vi "SW_Generate_Segmented_Plot_v2.vi"(0 "Draw Area Size":cluster{"Width":dbl, "Height":dbl}={"Width"=480.0, "Height"=480.0}, 1 "Input cluster of parameters":T1={"Amount of border segments"=8, "Border segments starting angle"=0, "Amount of midfield segments"=4, "Midfield segments starting angle"=0, "Midfield segments outer radius, mm"=60, "Amount of central segments"=1, "Center segment outer radius, mm"=30}, 2 "Diameter of the cage, mm":u16(knob)=180 scale=20.0..250.0, 3 "R-gap between segments, mm":u8=10, 4 "Colors array for outer segments":u32[](array[numeric])=[14102567, 16625249, 14742520, 7646673, 16018755, 16703632, 11262441, 4552116], 5 "Error In":errorcluster, 6 "Regions to mark":u16[](array[numeric]), 7 "Colors array for midfield segments":u32[](array[numeric])=[8073876, 10935200, 34871, 12756431], 9 "Color for central segment":u32=16777113) -> (12 "No zones Display output":picture, 14 "Zones Display output":picture, 15 "Actual parameters output":T4, 16 "Array of the segment to color correspondences":u32[][](array[numeric]), 17 "Array of the pixel to color correspondences":u32[][](array[numeric]), 18 "Pixels per mm":dbl=2.533333333333333, 19 "Error Out":errorcluster)   [LabVIEW 2016]
panel:
  out "Fonts scale factor":dbl
  out "Coordinates of the center of the image":T2
  out "Center segments outer radius, pix":dbl
  out "Midfield segments outer radius, pix":dbl
  out "Bounding rectangle of the midfield segments":T3
  out "Bounding rectangle for outer segments":T3
  in  "Fill color for no segments image":u32(colorbox)=6316128
  out "Radius of displayed outer segments, pix":dbl=228.0
  in  "Background color":u32(colorbox)=13816530
  in  "Zones Display input":picture
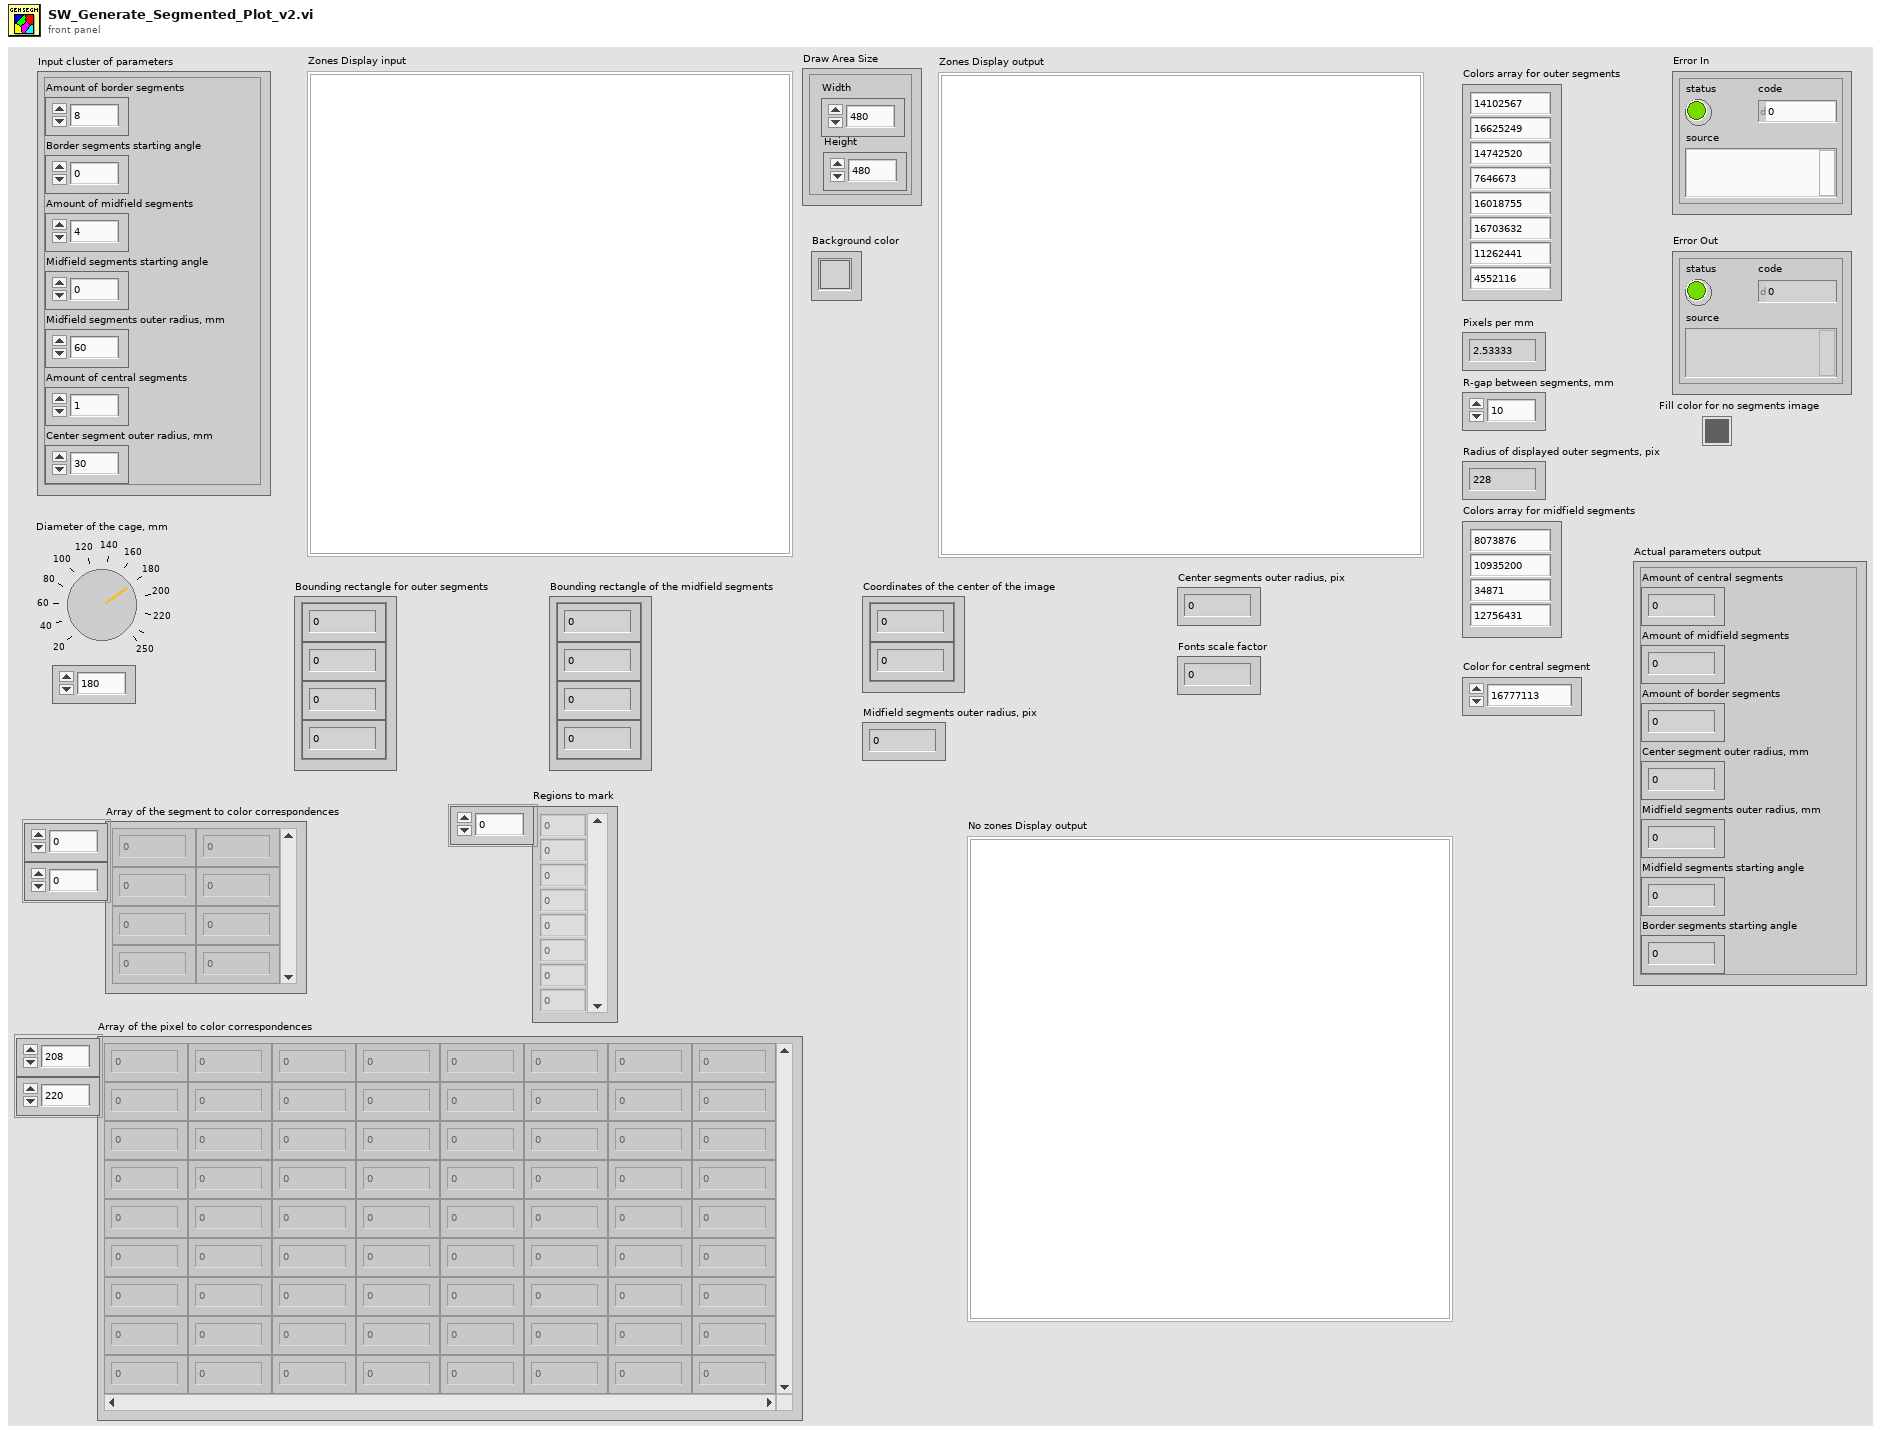
[diagram p1: front panel]
types:
  T1 = cluster{"Amount of border segments":u8, "Border segments starting angle":i16, "Amount of midfield segments":u8, "Midfield segments starting angle":i16, "Midfield segments outer radius, mm":u16, "Amount of central segments":u8, "Center segment outer radius, mm":u16}
  T2 = cluster{"Numeric Control":dbl, "Numeric Control":dbl}
  T3 = cluster{"Numeric Control":dbl, "Numeric Control":dbl, "Numeric Control":dbl, "Numeric Control":dbl}
  T4 = cluster{"Amount of central segments":u8, "Amount of midfield segments":u8, "Amount of border segments":u8, "Center segment outer radius, mm":u16, "Midfield segments outer radius, mm":u16, "Midfield segments starting angle":i16, "Border segments starting angle":i16}
  T5 = enum16{"User-specified Font", "Application Font", "System Font", "Dialog Font"}
  T6 = cluster{"horizontal":enum16{"left", "center", "right"}, "vertical":enum16{"top", "center", "bottom"}}
  T7 = cluster{"Width":u16, "Style":enum32{"Solid", "Dash", "Dot", "DashDot", "DashDotDot"}}
  T8 = cluster{"Amount of central segments":u8, "Amount of midfield segments":u8, "Amount of border segments":u8, u16, u16, i16, i16}
  T9 = typedef "imagedata.ctl" = cluster{"image type":i32, "image depth":i32, "image":u8[], "mask":u8[], "colors":u32[], "Rectangle":cluster{"left":i16, "top":i16, "right":i16, "bottom":i16}}
  T10 = cluster{"left":i16, "top":i16, "right":i16, "bottom":i16}
  T11 = cluster{"image[0]":u8, "image[1]":u8, "image[2]":u8}
  T12 = cluster{"Font Name:":string, "Size":i16, "Strikeout?":bool, "Italic?":bool, "Underline?":bool, "Outline?":bool, "Shadow?":bool, "Bold?":bool}
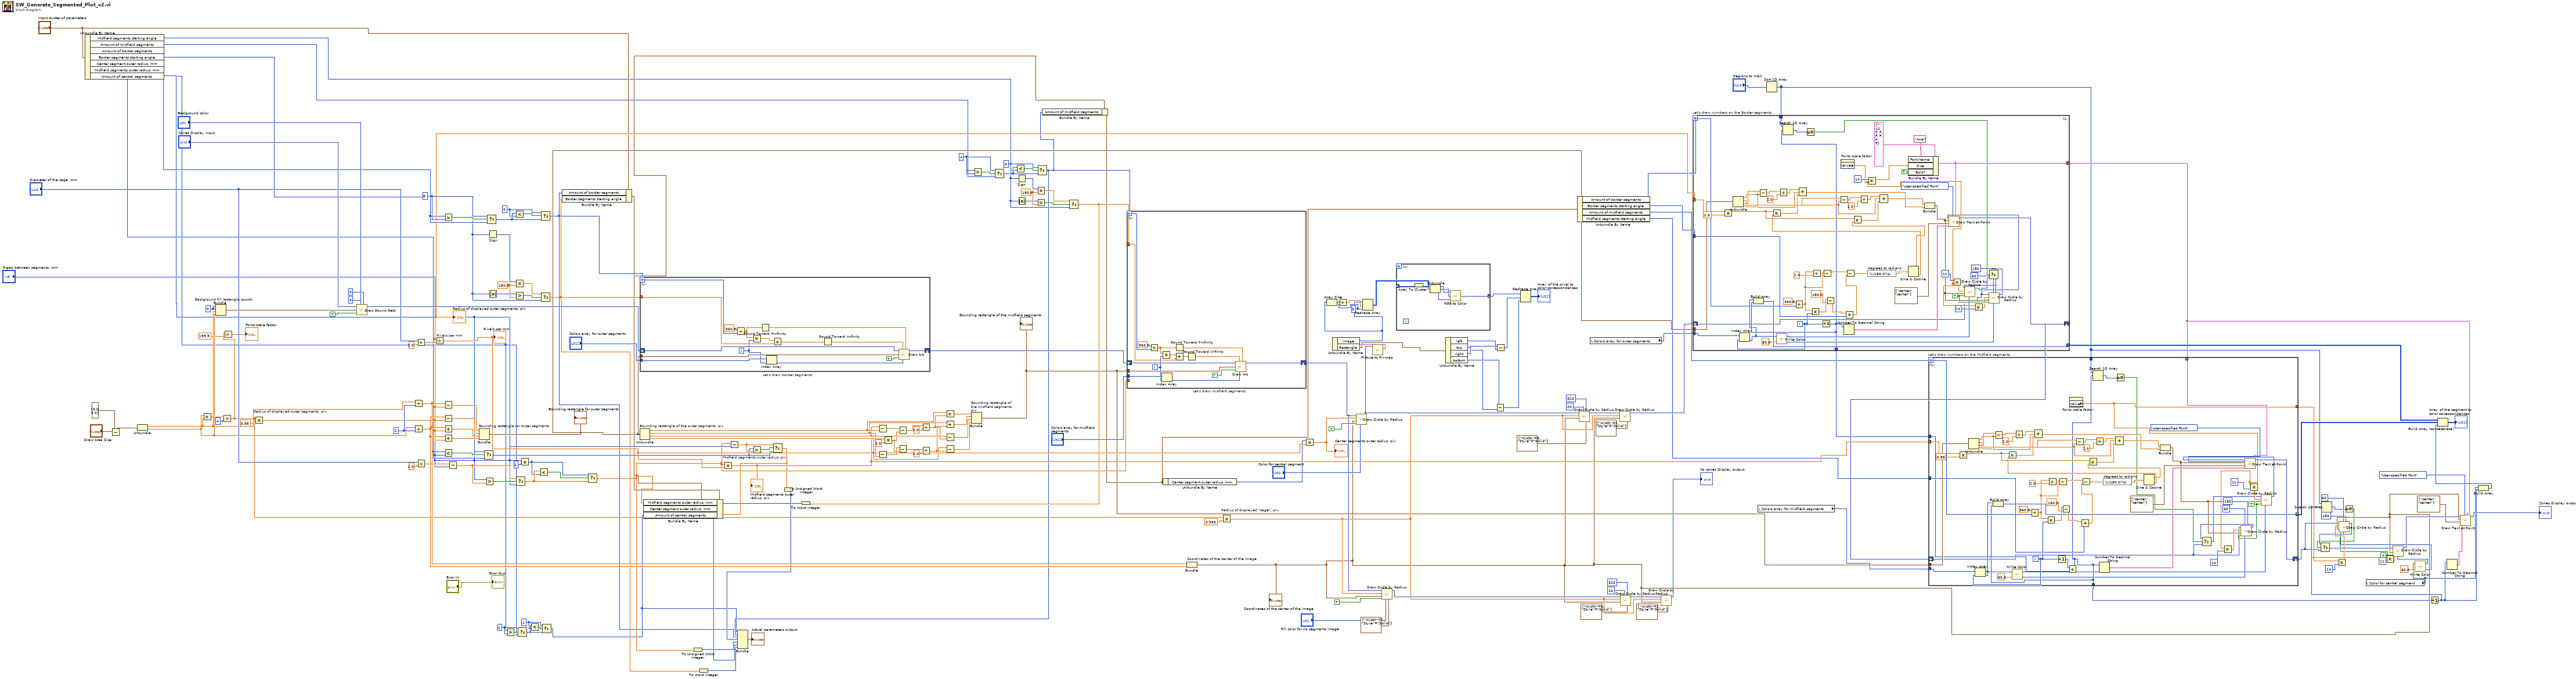
[diagram p0: block diagram]
diagram:
  w59 = 3 ("dimension size")
  w5 = TRUE ("fill?(F)")
  w146 = 180.0 ("y")
  w152 = u8 1 ("y")
  w149 = u8 1 ("y")
  w153 = u8 4 ("y")
  w156 = u8 0 ("y")
  w176 = u8 0 ("y")
  w178 = u8 8 ("y")
  w181 = 180.0 ("y")
  w190 = u32 2 ("y")
  w192 = 0
  n1 = Unbundle By Name("Input cluster of parameters") -> ("Midfield segments starting angle"=w29:i16, "Amount of midfield segments"=w28:u8, "Amount of border segments"=w27:u8, "Border segments starting angle"=w26:i16, "Center segment outer radius, mm"=w25:u16, "Midfield segments outer radius, mm"=w24:u16, "Amount of central segments"=w23:u8)
  n2 = Subtract(x="Draw Area Size", y=cluster{"Width":dbl, "Height":dbl} {"Width"=6.0, "Height"=6.0}) -> (x-y=w87:cluster{"Width":dbl, "Height":dbl})
  n3 = Unbundle(w87) -> ("Width"=w188:dbl, "Height"=w189:dbl)
  n4 = Add(x=w189, y=w188) -> (x+y=w187:dbl)
  n5 = Bundle "Background fill rectangle coords"(w192, w192, "Width"=w188, "Height"=w189) -> (w174:cluster{i32, i32, "Width":dbl, "Height":dbl})  [unwired: 1 in]
  n6 = Divide(x=w187, y=u32 4) -> (x/y=w22:dbl)
  n7 = Divide(x=w22, y=199.5) -> (x/y=→"Fonts scale factor":dbl)
  n8 = Multiply "Radius of displayed outer segments, pix"(x=w22, y=0.95) -> (x*y=w71:dbl)
  "Radius of displayed outer segments, pix" <- w71
  n9 = call <vilib>:"Draw Round Rect.vi"("picture"="Zones Display input", "oval width"=i16 0, "rect"=w174, "fill?(F)"=TRUE, "color(black)"="Background color", "oval height"=i16 0) -> ("new picture"=w173:picture)  [unwired: 3 in]
  n10 = Divide(x=w188, y=w190) -> (x/y=w172:dbl)
  n11 = Divide(x=w189, y=w190) -> (x/y=w171:dbl)
  n12 = Divide(x="Diameter of the cage, mm", y=2.0) -> (x/y=w160:dbl)
  n13 = Divide(x="Diameter of the cage, mm", y=2.0) -> (x/y=w138:dbl)
  n14 = Divide "Pixels per mm"(x=w71, y=w160) -> (x/y=w100:dbl)
  "Pixels per mm" <- w100
  n15 = Greater?(x=w27, y=w178) -> (0:w179:bool)
  n16 = Subtract(x=w172, y=w71) -> (x-y=w170:dbl)
  n17 = Subtract(x=w171, y=w71) -> (x-y=w169:dbl)
  n18 = Add(x=w172, y=w71) -> (x+y=w168:dbl)
  n19 = Add(x=w171, y=w71) -> (x+y=w167:dbl)
  n20 = Less?(x=w25, y="R-gap between segments, mm") -> (x < y?=w136:bool)
  n21 = Subtract(x=w138, y="R-gap between segments, mm") -> (x-y=w141:dbl)
  n22 = Bundle "Bounding rectangle for outer segments"(w170, w169, w168, w167) -> (w72:cluster{dbl, dbl, dbl, dbl})  [unwired: 1 in]
  "Bounding rectangle for outer segments" <- w72
  n23 = Select(t="R-gap between segments, mm", s=w136, f=w25) -> (s? t:f=w133:u16)
  n24 = Greater?(x=w24, y=w141) -> (0:w142:bool)
  n25 = Select(t=w178, s=w179, f=w27) -> (s? t:f=w175:u8)
  n26 = Sign(1:w26) -> (0:w182:i16)
  n27 = Absolute Value(x=w26) -> (abs(x)=w184:i16)
  n28 = Greater?(x=w23, y=w152) -> (0:w151:bool)
  n29 = Less?(x=w175, y=w176) -> (x < y?=w177:bool)
  n30 = Multiply(x=w182, y=w181) -> (x*y=w180:dbl)
  n31 = Greater?(x=w184, y=w181) -> (0:w183:bool)
  n32 = Select(t=w141, s=w142, f=w24) -> (s? t:f=w139:dbl)
  n33 = Select(t=w152, s=w151, f=w23) -> (s? t:f=w148:u8)
  n34 = Multiply(x="R-gap between segments, mm", y=u8 2) -> (x*y=w132:u8)
  n35 = Less?(x=w148, y=w149) -> (x < y?=w150:bool)
  n36 = Less?(x=w139, y=w132) -> (x < y?=w140:bool)
  n37 = Select(t=w176, s=w177, f=w175) -> (s? t:f=w44:u8)
  n38 = Select(t=w180, s=w183, f=w26) -> (s? t:f=w43:dbl)
  n39 = Select(t=w149, s=w150, f=w148) -> (s? t:f=w37:u8)
  n40 = Bundle By Name(cluster="Input cluster of parameters", "Amount of border segments"=w44, "Border segments starting angle"=w43) -> (w41:T1)
  n41 = Select(t=w132, s=w140, f=w139) -> (s? t:f=w39:dbl)
  n42 = for "Let's draw border segments" {
    N: w44 -> [w203]
    tunnel: w43 -> [w208]
    shift-right: [w201] -> w158
    shift-left: w173 -> [w210]
    tunnel: w72 -> [w204]
    tunnel: "Colors array for outer segments" -> [w207]
    i -> [w198]
    n43 = Divide(x=360.0, y=w203) -> (x/y=w202:dbl)
    n44 = Multiply(x=w202, y=w198) -> (x*y=w209:dbl)
    n45 = Round Toward +Infinity(x=w202) -> (ceil(x): smallest int >= x=w200:dbl)
    n46 = Index Array(array=w207, index=w198) -> (element=w197:u32)
    n47 = Add(x=w209, y=w208) -> (x+y=w205:dbl)
    n48 = Round Toward -Infinity(1:w205) -> (0:w199:dbl)
    n49 = call <vilib>:"Draw Arc.vi"("picture"=w210, "start angle[degrees]"=w199, "rect"=w204, "fill?(F)"=TRUE, "color(black)"=w197, "arc size[degrees]"=w200) -> ("new picture"=w201:picture)  [unwired: 3 in]
  }
  n50 = Unbundle "Bounding rectangle of the outer segments, pix"(w72) -> (w126:dbl, w118:dbl, w124:dbl, w117:dbl)
  n51 = To Unsigned Word Integer(number=w39) -> (unsigned 16bit integer=w105:u16)
  n52 = To Word Integer(number=w43) -> (16bit integer=w101:i16)
  n53 = Multiply "Midfield segments outer radius, pix"(x=w39, y=w100) -> (x*y=w69:dbl)
  "Midfield segments outer radius, pix" <- w69
  n54 = Subtract(x=w39, y="R-gap between segments, mm") -> (x-y=w134:dbl)
  n55 = Greater?(x=w133, y=w134) -> (0:w135:bool)
  n56 = Select(t=w134, s=w135, f=w133) -> (s? t:f=w38:dbl)
  n57 = Bundle By Name(cluster=w41, "Midfield segments outer radius, mm"=w39, "Center segment outer radius, mm"=w38, "Amount of central segments"=w37) -> (w40:T1)
  n58 = To Unsigned Word Integer(number=w38) -> (unsigned 16bit integer=w103:u16)
  n59 = Subtract(x=w124, y=w126) -> (x-y=w130:dbl)
  n60 = Subtract(x=w117, y=w118) -> (x-y=w123:dbl)
  n61 = Multiply(x=w69, y=2.0) -> (x*y=w122:dbl)
  n62 = Subtract(x=w130, y=w122) -> (x-y=w128:dbl)
  n63 = Subtract(x=w123, y=w122) -> (x-y=w120:dbl)
  n64 = Divide(x=w128, y=2.0) -> (x/y=w125:dbl)
  n65 = Divide(x=w120, y=2.0) -> (x/y=w119:dbl)
  n66 = Add(x=w126, y=w125) -> (x+y=w116:dbl)
  n67 = Add(x=w118, y=w119) -> (x+y=w114:dbl)
  n68 = Subtract(x=w124, y=w125) -> (x-y=w115:dbl)
  n69 = Subtract(x=w117, y=w119) -> (x-y=w113:dbl)
  n70 = Bundle "Bounding rectangle of the midfield segments, pix"(w116, w114, w115, w113) -> (w70:cluster{dbl, dbl, dbl, dbl})  [unwired: 1 in]
  "Bounding rectangle of the midfield segments" <- w70
  n71 = Greater?(x=w28, y=w153) -> (0:w154:bool)
  n72 = Select(t=w153, s=w154, f=w28) -> (s? t:f=w157:u8)
  n73 = Less?(x=w157, y=w156) -> (x < y?=w155:bool)
  n74 = Sign(1:w29) -> (0:w145:i16)
  n75 = Absolute Value(x=w29) -> (abs(x)=w143:i16)
  n76 = Multiply(x=w145, y=w146) -> (x*y=w147:dbl)
  n77 = Greater?(x=w143, y=w146) -> (0:w144:bool)
  n78 = Select(t=w156, s=w155, f=w157) -> (s? t:f=w42:u8)
  n79 = Bundle By Name(cluster=w40, "Amount of midfield segments"=w42) -> (w35:T1)
  n80 = Select(t=w147, s=w144, f=w29) -> (s? t:f=w104:dbl)
  n81 = To Word Integer(number=w104) -> (16bit integer=w102:i16)
  n82 = Bundle("Amount of central segments"=w37, "Amount of midfield segments"=w42, "Amount of border segments"=w44, w103, w105, w102, w101) -> (→"Actual parameters output":T8)  [unwired: 1 in]
  n83 = for "Let's draw midfield segments" {
    N: w42 -> [w217]
    shift-right: [w212] -> w93
    shift-left: w158 -> [w213]
    tunnel: w104 -> [w215]
    tunnel: w39 -> [_]
    tunnel: w70 -> [w214]
    tunnel: "Colors array for midfield segments" -> [w219]
    i -> [w216]
    n84 = Divide(x=360.0, y=w217) -> (x/y=w221:dbl)
    n85 = Multiply(x=w221, y=w216) -> (x*y=w222:dbl)
    n86 = Index Array(array=w219, index=w216) -> (element=w218:u32)
    n87 = Round Toward +Infinity(x=w221) -> (ceil(x): smallest int >= x=w224:dbl)
    n88 = Add(x=w222, y=w215) -> (x+y=w223:dbl)
    n89 = Round Toward -Infinity(1:w223) -> (0:w225:dbl)
    n90 = call <vilib>:"Draw Arc.vi"("picture"=w213, "start angle[degrees]"=w225, "rect"=w214, "fill?(F)"=TRUE, "color(black)"=w218, "arc size[degrees]"=w224) -> ("new picture"=w212:picture)  [unwired: 3 in]
  }
  n91 = Unbundle By Name(w35) -> ("Center segment outer radius, mm"=w36:u16)
  n92 = Bundle "Coordinates of the center of the image"(w172, w171) -> (w9:cluster{dbl, dbl})  [unwired: 1 in]
  "Coordinates of the center of the image" <- w9
  n93 = Multiply "Radius of displayed \"cage\", pix"(x=w22, y=0.955) -> (x*y=w89:dbl)
  n94 = Multiply(x=w36, y=w100) -> (x*y=w109:dbl)
  "Center segments outer radius, pix" <- w109
  n95 = call <vilib>:"Draw Circle by Radius.vi"("color(black)"="Color for central segment", "fill?(F)"=TRUE, "pixel center"=w9, "radius"=w109, "picture"=w93) -> ("new picture"=w63:picture)  [unwired: 6 in]
  n96 = call <vilib>:"Picture to Pixmap.vi"("picture"=w63) -> ("image data"=w62:T9)  [unwired: 9 in, 1 out]
  n97 = Unbundle By Name(w62) -> ("image"=w61:u8[], "Rectangle"=w56:T10)
  n98 = Array Size(array=w61) -> (size(s)=w60:i32)
  n99 = Divide(x=w60, y=w59) -> (x/y=w58:dbl)
  n100 = Reshape Array(w61, w58, w59) -> (w57:u8[][])
  n101 = call <vilib>:"Draw Circle by Radius.vi"("pen"=T7 {"Width"=2, "Style"=enum."Solid"}, "color(black)"="Fill color for no segments image", "fill?(F)"=TRUE, "pixel center"=w9, "radius"=w89, "picture"=w93) -> ("new picture"=w90:picture)  [unwired: 5 in]
  n102 = for {
    tunnel: w57 -> [w232] mode=indexing
    tunnel: [w227] -> w55 mode=indexing
    n103 = Array To Cluster(array=w232) -> (cluster=w231:T11)
    n104 = Unbundle(w231) -> ("image[0]"=w230:u8, "image[1]"=w229:u8, "image[2]"=w228:u8)
    n105 = call <vilib>:"RGB to Color.vi"("B"=w228, "G"=w229, "R"=w230) -> ("Color"=w227:u32)
  }
  n106 = Unbundle By Name(w56) -> ("left"=w53:i16, "top"=w50:i16, "right"=w54:i16, "bottom"=w51:i16)
  n107 = Subtract(x=w51, y=w50) -> (x-y=w49:i16)
  n108 = Subtract(x=w54, y=w53) -> (x-y=w52:i16)
  n109 = Reshape Array(w55, w52, w49) -> (→"Array of the pixel to color correspondences":u32[][])
  n110 = Unbundle By Name(w35) -> ("Amount of border segments"=w34:u8, "Border segments starting angle"=w33:i16, "Amount of midfield segments"=w32:u8, "Midfield segments starting angle"=w31:i16)
  n111 = call <vilib>:"Draw Circle by Radius.vi"("pen"=T7 {"Width"=6, "Style"=enum."Solid"}, "arc size(360)"=i16 320, "start angle(0)"=i16 20, "pixel center"=w9, "radius"=w89, "picture"=w63) -> ("new picture"=w166:picture)  [unwired: 5 in]
  n112 = local read "Colors array for outer segments"() -> (w82:u32[])
  n113 = call <vilib>:"Draw Circle by Radius.vi"("pen"=T7 {"Width"=2, "Style"=enum."Solid"}, "pixel center"=w9, "radius"=w89, "picture"=w166) -> ("new picture"=w84:picture)  [unwired: 7 in]
  n114 = call <vilib>:"Draw Circle by Radius.vi"("pen"=T7 {"Width"=6, "Style"=enum."Solid"}, "arc size(360)"=i16 320, "start angle(0)"=i16 20, "pixel center"=w9, "radius"=w89, "picture"=w90) -> ("new picture"=w94:picture)  [unwired: 5 in]
  n115 = call <vilib>:"Draw Circle by Radius.vi"("pen"=T7 {"Width"=2, "Style"=enum."Solid"}, "pixel center"=w9, "radius"=w89, "picture"=w94) -> ("new picture"=→"No zones Display output":picture)  [unwired: 7 in]
  n116 = local read "Colors array for midfield segments"() -> (w81:u32[])
  n117 = Sort 1D Array(array="Regions to mark") -> (sorted array=w13:u16[])
  n118 = for "Let's draw numbers on the Border segments" {
    N: w34 -> [w297]
    tunnel: w33 -> [w298]
    shift-right: [w277] -> w83
    shift-left: w84 -> [w237]
    tunnel: w72 -> [w292]
    tunnel: w82 -> [w265]
    tunnel: w71 -> [w261]
    tunnel: [w248] -> w80
    tunnel: [w258] -> w67 mode=indexing
    tunnel: [w250] -> w19
    tunnel: w13 -> [w249]
    i -> [w264]
    w243 = TRUE ("fill?(F)")
    n119 = Multiply(x=w261, y=0.9) -> (x*y=w260:dbl)
    n120 = Unbundle(w292) -> (w286:dbl, w279:dbl, w291:dbl, w278:dbl)
    n121 = Index Array(array=w265, index=w264) -> (element=w234:u32)
    n122 = Subtract(x=w291, y=w286) -> (x-y=w289:dbl)
    n123 = call <vilib>:"Hilite Color.vi"("Percentage(30)"=60.0, "Color In"=w234) -> ("Shadow"=w233:u32, "Hilite"=w263:u32)
    n124 = Divide(x=w289, y=2.0) -> (x/y=w287:dbl)
    n125 = Divide(x=360.0, y=w297) -> (x/y=w267:dbl)
    n126 = Multiply(x=w267, y=w264) -> (x*y=w271:dbl)
    n127 = Divide(x=w267, y=2.0) -> (x/y=w269:dbl)
    n128 = Increment(x=w264) -> (x+1=w248:i32)
    n129 = Build Array(w234, w248) -> (w258:u32[])
    n130 = Search 1D Array(1D array=w249, element=w248) -> (index of element=w247:i32)  [unwired: 1 in]
    n131 = Greater Or Equal To 0?(x=w247) -> (x >= 0?=w246:bool)
    n132 = Subtract(x=w269, y=w267) -> (x-y=w268:dbl)
    n133 = Subtract(x=w271, y=180.0) -> (x-y=w272:dbl)
    n134 = Subtract(x=w278, y=w279) -> (x-y=w281:dbl)
    n135 = property on="Fonts scale factor" class="DigNum (strict)"() -> ("Value"=w242:dbl)  [unwired: 2 in, 2 out]
    n136 = Number To Decimal String(number=w248) -> (decimal integer string=w275:string)  [unwired: 1 in]
    n137 = Add(x=w272, y=w298) -> (x+y=w295:dbl)
    n138 = Subtract(x=w268, y=w295) -> (x-y=w294:dbl)
    n139 = Divide(x=w281, y=2.0) -> (x/y=w283:dbl)
    n140 = Multiply(x=i16 14 ("Size"), y=w242) -> (x*y=w252:dbl)
    n141 = expression code="(x/180.0)*pi" "degrees to radians"(w294) -> (w293:dbl)
    n142 = Bundle By Name(cluster=T12 {"Font Name:"="", "Size"=12, "Strikeout?"=FALSE, "Italic?"=FALSE, "Underline?"=FALSE, "Outline?"=FALSE, "Shadow?"=FALSE, "Bold?"=FALSE} ("[user-specified font]"), "Font Name:"="Arial", "Size"=w252, "Bold?"=TRUE) -> (w250:T12)
    n143 = Sine & Cosine(0:w293) -> (1:w280:dbl, 2:w290:dbl)
    n144 = Multiply(x=w260, y=w290) -> (x*y=w285:dbl)
    n145 = Compound Arithmetic op=ADD(w287, w286, w285) -> (w274:dbl)
    n146 = Multiply(x=w260, y=w280) -> (x*y=w284:dbl)
    n147 = Compound Arithmetic op=ADD(w283, w279, w284) -> (w273:dbl)
    n148 = Bundle(w273, w274) -> (w244:cluster{dbl, dbl})  [unwired: 1 in]
    n149 = Multiply(x=i16 11 ("radius"), y=w242) -> (x*y=w251:dbl)
    n150 = Multiply(x=w242, y=14) -> (x*y=w240:dbl)
    n151 = call <vilib>:"Draw Circle by Radius.vi"("arc size(360)"=i16 180, "color(black)"=w233, "start angle(0)"=i16 60, "fill?(F)"=w243, "pixel center"=w244, "radius"=w240, "picture"=w237) -> ("new picture"=w245:picture)  [unwired: 4 in]
    n152 = Select(t=w245, s=w246, f=w237) -> (s? t:f=w236:picture)
    n153 = call <vilib>:"Draw Circle by Radius.vi"("color(black)"=w263, "fill?(F)"=w243, "pixel center"=w244, "radius"=w251, "picture"=w236) -> ("new picture"=w235:picture)  [unwired: 6 in]
    n154 = call <vilib>:"Draw Text at Point.vi"("[user-specified font]"=w250, "desired font(Application)"=T5."User-specified Font", "text"=w275, "alignment(left, top)"=T6 {"horizontal"=enum."center", "vertical"=enum."center"}, "origin"=w244, "picture"=w235) -> ("new picture"=w277:picture)  [unwired: 4 in, 1 out]
  }
  n155 = for "Let's draw numbers on the Midfield segments" {
    N: w32 -> [w361]
    tunnel: w31 -> [w362]
    shift-right: [w340] -> w11
    shift-left: w83 -> [w309]
    tunnel: w70 -> [w356]
    tunnel: w81 -> [w324]
    tunnel: w69 -> [w343]
    tunnel: w80 -> [w320]
    tunnel: [w312] -> w73
    tunnel: [w318] -> w66 mode=indexing
    tunnel: w19 -> [w315]
    tunnel: [w300] -> w7
    tunnel: w13 -> [w313]
    i -> [w323]
    w305 = TRUE ("fill?(F)")
    n156 = Multiply(x=w343, y=0.85) -> (x*y=w337:dbl)
    n157 = Unbundle(w356) -> (w350:dbl, w342:dbl, w355:dbl, w341:dbl)
    n158 = Index Array(array=w324, index=w323) -> (element=w319:u32)
    n159 = Subtract(x=w355, y=w350) -> (x-y=w353:dbl)
    n160 = call <vilib>:"Hilite Color.vi"("Percentage(30)"=60.0, "Color In"=w319) -> ("Shadow"=w303:u32, "Hilite"=w322:u32)
    n161 = Divide(x=w353, y=2.0) -> (x/y=w351:dbl)
    n162 = Divide(x=360.0, y=w361) -> (x/y=w327:dbl)
    n163 = Multiply(x=w327, y=w323) -> (x*y=w332:dbl)
    n164 = Divide(x=w327, y=2.0) -> (x/y=w329:dbl)
    n165 = Increment(x=w323) -> (x+1=w330:i32)
    n166 = Subtract(x=w329, y=w327) -> (x-y=w328:dbl)
    n167 = Subtract(x=w332, y=180.0) -> (x-y=w333:dbl)
    n168 = Add(x=w330, y=w320) -> (x+y=w312:i32)
    n169 = Build Array(w319, w312) -> (w318:u32[])
    n170 = property on="Fonts scale factor" class="DigNum (strict)"() -> ("Value"=w300:dbl)  [unwired: 2 in, 2 out]
    n171 = Subtract(x=w341, y=w342) -> (x-y=w345:dbl)
    n172 = Add(x=w333, y=w362) -> (x+y=w359:dbl)
    n173 = Subtract(x=w328, y=w359) -> (x-y=w358:dbl)
    n174 = Search 1D Array(1D array=w313, element=w312) -> (index of element=w314:i32)  [unwired: 1 in]
    n175 = Divide(x=w345, y=2.0) -> (x/y=w347:dbl)
    n176 = Number To Decimal String(number=w312) -> (decimal integer string=w338:string)  [unwired: 1 in]
    n177 = expression code="(x/180.0)*pi" "degrees to radians"(w358) -> (w357:dbl)
    n178 = Greater Or Equal To 0?(x=w314) -> (x >= 0?=w311:bool)
    n179 = Sine & Cosine(0:w357) -> (1:w344:dbl, 2:w354:dbl)
    n180 = Multiply(x=w337, y=w354) -> (x*y=w349:dbl)
    n181 = Compound Arithmetic op=ADD(w351, w350, w349) -> (w335:dbl)
    n182 = Multiply(x=w337, y=w344) -> (x*y=w348:dbl)
    n183 = Compound Arithmetic op=ADD(w347, w342, w348) -> (w334:dbl)
    n184 = Bundle(w334, w335) -> (w304:cluster{dbl, dbl})  [unwired: 1 in]
    n185 = Multiply(x=w300, y=i16 14 ("radius")) -> (x*y=w301:dbl)
    n186 = call <vilib>:"Draw Circle by Radius.vi"("arc size(360)"=i16 180, "color(black)"=w303, "start angle(0)"=i16 60, "fill?(F)"=w305, "pixel center"=w304, "radius"=w301, "picture"=w309) -> ("new picture"=w308:picture)  [unwired: 4 in]
    n187 = Select(t=w308, s=w311, f=w309) -> (s? t:f=w310:picture)
    n188 = Multiply(x=w300, y=i16 11 ("radius")) -> (x*y=w316:dbl)
    n189 = call <vilib>:"Draw Circle by Radius.vi"("color(black)"=w322, "fill?(F)"=w305, "pixel center"=w304, "radius"=w316, "picture"=w310) -> ("new picture"=w325:picture)  [unwired: 6 in]
    n190 = call <vilib>:"Draw Text at Point.vi"("[user-specified font]"=w315, "desired font(Application)"=T5."User-specified Font", "text"=w338, "alignment(left, top)"=T6 {"horizontal"=enum."center", "vertical"=enum."center"}, "origin"=w304, "picture"=w325) -> ("new picture"=w340:picture)  [unwired: 4 in, 1 out]
  }
  n191 = Multiply(x=w7, y=i16 14 ("radius")) -> (x*y=w6:dbl)
  n192 = local read "Color for central segment"() -> (w68:u32)
  n193 = Multiply(x=w7, y=i16 11 ("radius")) -> (x*y=w17:dbl)
  n194 = call <vilib>:"Hilite Color.vi"("Percentage(30)"=60.0, "Color In"=w68) -> ("Shadow"=w4:u32, "Hilite"=w78:u32)
  n195 = call <vilib>:"Draw Circle by Radius.vi"("arc size(360)"=i16 180, "color(black)"=w4, "start angle(0)"=i16 60, "fill?(F)"=w5, "pixel center"=w9, "radius"=w6, "picture"=w11) -> ("new picture"=w10:picture)  [unwired: 4 in]
  n196 = Increment(x=w73) -> (x+1=w12:i32)
  n197 = Search 1D Array(1D array=w13, element=w12) -> (index of element=w14:i32)  [unwired: 1 in]
  n198 = Greater Or Equal To 0?(x=w14) -> (x >= 0?=w1:bool)
  n199 = Select(t=w10, s=w1, f=w11) -> (s? t:f=w15:picture)
  n200 = call <vilib>:"Draw Circle by Radius.vi"("color(black)"=w78, "fill?(F)"=w5, "pixel center"=w9, "radius"=w17, "picture"=w15) -> ("new picture"=w76:picture)  [unwired: 6 in]
  n201 = Number To Decimal String(number=w12) -> (decimal integer string=w74:string)  [unwired: 1 in]
  n202 = call <vilib>:"Draw Text at Point.vi"("[user-specified font]"=w19, "desired font(Application)"=T5."User-specified Font", "text"=w74, "alignment(left, top)"=T6 {"horizontal"=enum."center", "vertical"=enum."center"}, "origin"=w9, "picture"=w76) -> ("new picture"=→"Zones Display output":picture)  [unwired: 4 in, 1 out]
  n203 = Build Array(w68, w12) -> (w65:u32[])
  n204 = Build Array (concatenate)(w67, w66, w65) -> (→"Array of the segment to color correspondences":u32[][])
  "Error Out" <- "Error In"
